vi "RegisteredMessages.vi"() -> (3 "registered messages":string[](array[string]))   [LabVIEW 2017, in "EmsaAcquisition.lvlib"]
uses:
  <vilib>/addons/InsightCM/Devices/Shared/Emsa/EmsaAcquisition/EmsaAcquisition.lvlib
  <vilib>/addons/InsightCM/Devices/Shared/Common/FpgaBitfileManager/FpgaBitfileManager.lvlib
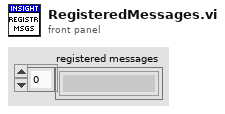
[diagram p1: front panel]
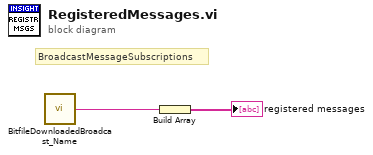
[diagram p0: block diagram]
diagram:
  # "BroadcastMessageSubscriptions"
  n1 = call <vilib>:"BitfileDownloadedBroadcast_Name.vi"() -> ("message name"=w1:string)  [unwired: 5 in]
  n2 = Build Array(w1) -> (→"registered messages":string[])
